vi "Add Menu Item.vi"(8 "error in (no error)":errorcluster, 9 "Reset":bool, 10 "Item Names":string[](array[string]), 11 "Queed Listbox ref":refnum<vi>) -> (0 "error out":errorcluster, 2 "Current Strings":string[](array[string]), 3 "Queed Listbox ref out":refnum<vi>)   [LabVIEW 2015]
uses:
  Queued Listbox.xctl
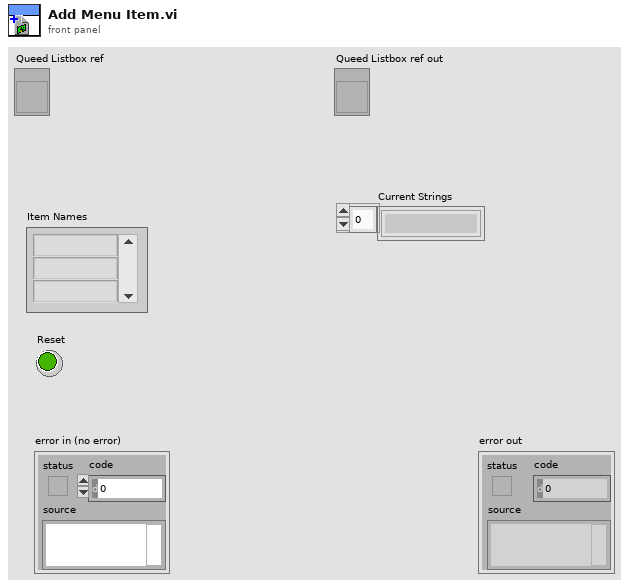
[diagram p1: front panel]
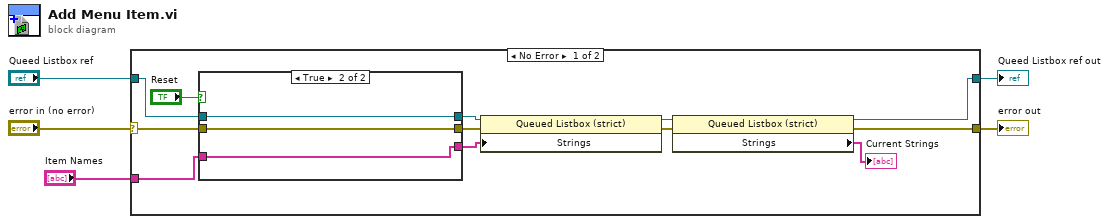
[diagram p0: block diagram]
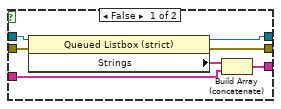
[diagram p2: hidden frame]
diagram:
  n1 = case shown="No Error" "error in (no error)" {
    selector: "error in (no error)" -> [w15 w29]
    tunnel: [w10 w29] -> w3
    tunnel: "Item Names" -> [w16 _]
    tunnel: "Queed Listbox ref" -> [w8 w28]
    tunnel: [w7 w28] -> w1
    frame No Error {
      n2 = case shown="True" "Reset" {
        tunnel: [w24 w25] -> w17
        tunnel: w16 -> [w22 w27]
        tunnel: w15 -> [w21 w26]
        tunnel: [w20 w26] -> w14
        tunnel: [w19 w27] -> w13
        tunnel: w8 -> [w18 w25]
        frame False {
          n3 = property class="Queued Listbox (strict)"(reference=w18, error in=w21) -> (reference out=w24:refnum<vi>, error out=w20:errorcluster, "Strings"=w23:string[])
          n4 = Build Array (concatenate)(w23, w22) -> (w19:string[])
        }
        frame True {
        }
      }
      n5 = property class="Queued Listbox (strict)"(reference=w17, error in=w14, "Strings"=w13) -> (reference out=w11:refnum<vi>, error out=w12:errorcluster)
      n6 = property class="Queued Listbox (strict)"(reference=w11, error in=w12) -> (reference out=w7:refnum<vi>, error out=w10:errorcluster, "Strings"=→"Current Strings":string[])
    }
    frame Error {
    }
  }
  "error out" <- w3
  "Queed Listbox ref out" <- w1
